vi "Check Disabled.vi"(8 "error in (no error)":errorcluster, 10 "Array":T1(array[cluster]), 11 "LoggingControl in":refnum<class "GroupLoggingControl.lvclass">) -> (0 "error out":errorcluster, 3 "LoggingControl out":refnum<class "GroupLoggingControl.lvclass">)   [LabVIEW 2020, in "VolatusGUIElements.lvlib" / "GroupLoggingControl.lvclass"]
uses:
  GroupLoggingControl.lvclass
  GroupLoggingControl.lvclass/GroupLoggingControl.ctl
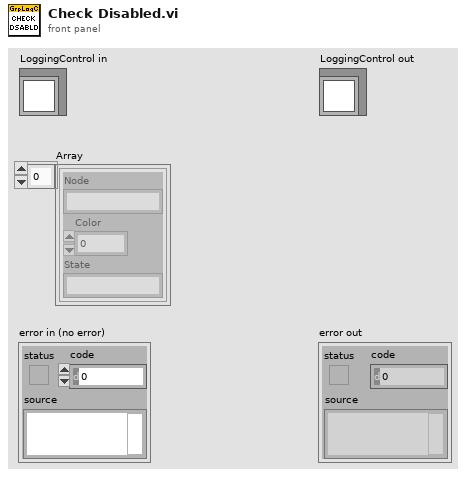
[diagram p1: front panel]
types:
  T1 = cluster{"Node":string, "Color":u32, "State":string}[]
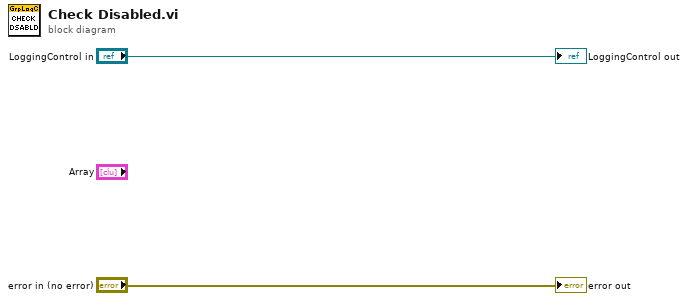
[diagram p0: block diagram]
diagram:
  "error out" <- "error in (no error)"
  "LoggingControl out" <- "LoggingControl in"
